vi "A33ConfigurePulse_py.vi"(5 "Trailing edge":dbl=4e-09 format="%#_12g", 6 "Pulse width":dbl=0.1 format="%#_12g", 7 "Leading edge":dbl=4e-09 format="%#_12g", 9 "Pulse period":dbl=1.0 format="%#_12g") -> ()   [LabVIEW 2022 SP3]
doc: "Selects the waveform shape, frequency, amplitude, offset, and phase for a standard waveform."
uses:
  <vilib>/addons/zeromq/zmq_socket.lvclass
panel:
  in  "Channel (1: Channel1)":i32(ring)=1 items=["Channel1"=1, "Channel2"=2]
  out "Standalone":bool
  out "socket out":refnum<class "zmq_socket.lvclass">
  in  "socket in":refnum<class "zmq_socket.lvclass">
  out "error out":errorcluster
  out "resulting string":string
  in  "Instrument":string="AG33600A_Gen1"
  in  "error in (no error)":errorcluster
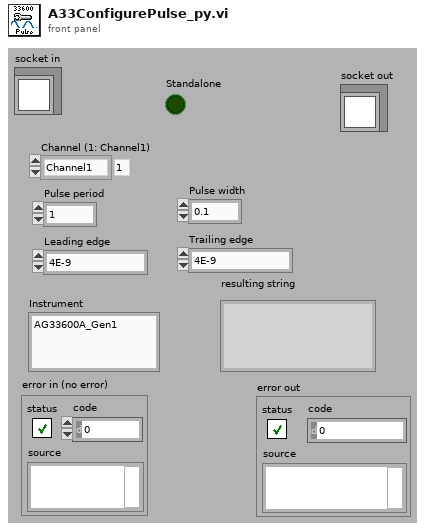
[diagram p1: front panel]
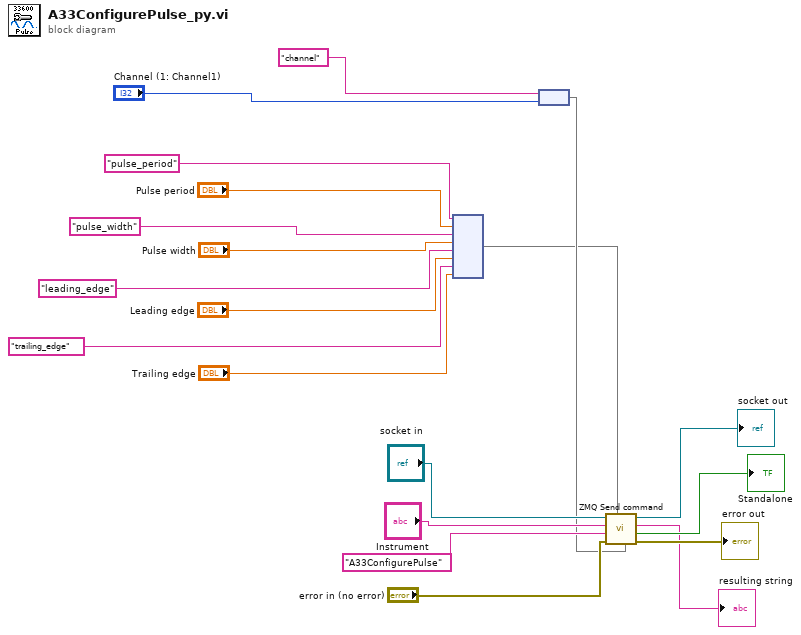
[diagram p0: block diagram]
diagram:
  n1 = node("pulse_period" ("key"), "Pulse period", "pulse_width" ("key"), "Pulse width", "leading_edge" ("key"), "Leading edge", "trailing_edge" ("key"), "Trailing edge") -> (w5:map{string, dbl})
  n2 = node("channel" ("key"), "Channel (1: Channel1)") -> (w6:map{string, i32})
  n3 = call "ZMQ Send command.vi"("Int args"=w6, "DBL args"=w5, "error in"="error in (no error)", "Command"="A33ConfigurePulse", "Instrument"="Instrument", "socket in"="socket in") -> ("error out"=→"error out":errorcluster, "Standalone"=→"Standalone":bool, "Recieved message"=→"resulting string":string, "socket out"=→"socket out":refnum<class "zmq_socket.lvclass">)  [unwired: 2 in]
